vi "subsystem manager fg.vi"(0 "Menu":T1, 1 "Ball State Write":enum16{"no ball", "holding", "loaded"}(ring), 2 "Picked Up":bool, 3 "Loaded":bool, 4 "Shooter Cocked":bool, 5 "Re-Initalize":bool, 8 "Arm Ready":bool) -> (14 "Ball State Read":enum16{"no ball", "holding", "loaded"}(ring), 16 "Picked Up":bool, 17 "Loaded":bool, 18 "Shooter Cocked":bool, 19 "Arm Ready":bool)   [LabVIEW 2013]
uses:
  typedefs/fg_typedef.ctl
panel:
  # "The Somewhat-Powerful Functional Global with a Bunch of the SubStates"
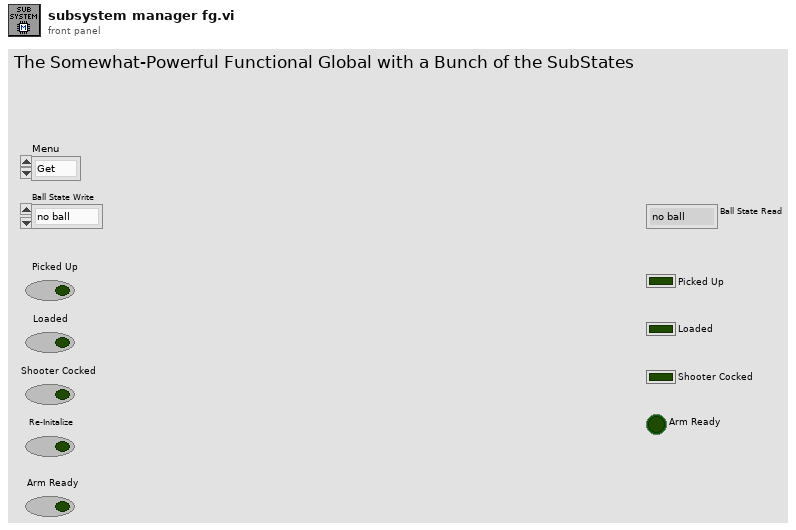
[diagram p1: front panel]
types:
  T1 = typedef "fg_typedef.ctl" = enum16{"Get", "Set"}
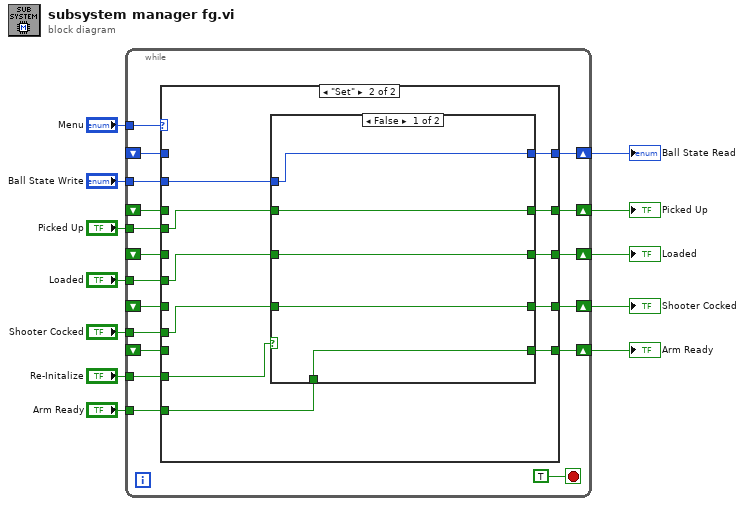
[diagram p0: block diagram]
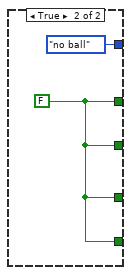
[diagram p3: hidden frame]
diagram:
  n1 = while {
    tunnel: "Menu" -> [w30]
    tunnel: "Ball State Write" -> [w29]
    shift-right: [w28] -> w10
    shift-left: _ -> [w27]
    shift-right: [w25] -> w6
    shift-left: _ -> [w24]
    tunnel: "Picked Up" -> [w23]
    shift-right: [w21] -> w8
    shift-left: _ -> [w20]
    tunnel: "Loaded" -> [w22]
    tunnel: "Shooter Cocked" -> [w19]
    shift-right: [w18] -> w4
    shift-left: _ -> [w17]
    tunnel: "Re-Initalize" -> [w16]
    tunnel: "Arm Ready" -> [w15]
    shift-right: [w14] -> w1
    shift-left: _ -> [w13]
    stop <- TRUE stop-if-true
    n2 = case shown="\"Set\"" w30 {
      tunnel: w29 -> [_ w39]
      tunnel: [w35 w38] -> w28
      tunnel: w27 -> [w35 _]
      tunnel: [w34 w40] -> w25
      tunnel: w24 -> [w34 _]
      tunnel: w23 -> [_ w41]
      tunnel: [w33 w42] -> w21
      tunnel: w22 -> [_ w43]
      tunnel: w20 -> [w33 _]
      tunnel: w19 -> [_ w45]
      tunnel: [w32 w44] -> w18
      tunnel: w17 -> [w32 _]
      tunnel: w16 -> [_ w46]
      tunnel: w15 -> [_ w37]
      tunnel: [w31 w36] -> w14
      tunnel: w13 -> [w31 _]
      frame "Get", Default {
      }
      frame "Set" {
        n3 = case shown="False" w46 {
          tunnel: w45 -> [w51 _]
          tunnel: [w51 w52] -> w44
          tunnel: w43 -> [w50 _]
          tunnel: [w50 w52] -> w42
          tunnel: w41 -> [w49 _]
          tunnel: [w49 w52] -> w40
          tunnel: w39 -> [w48 _]
          tunnel: [w48 enum16{"no ball", "holding", "loaded"}."no ball" ("Ball State Write")] -> w38
          tunnel: w37 -> [w47 _]
          tunnel: [w47 w52] -> w36
          frame False {
          }
          frame True {
            w52 = FALSE ("Picked Up")
          }
        }
      }
    }
  }
  "Ball State Read" <- w10
  "Picked Up" <- w6
  "Loaded" <- w8
  "Shooter Cocked" <- w4
  "Arm Ready" <- w1
